vi "Heartbeat Reset.vi"(8 "error in":errorcluster, 10 "CANopen Message":refnum<class "CANopen Response Message.lvclass">, 11 "CANopen Master in":refnum<class "CANopen Master.lvclass">) -> (0 "error out":errorcluster, 3 "CANopen Master out":refnum<class "CANopen Master.lvclass">)   [LabVIEW 2024, in "CANopen Master.lvlib" / "CANopen Master.lvclass"]
uses:
  CANopen Master.lvclass
  CANopen Master.lvclass/CANopen Master.ctl
  Heartbeat/Heartbeat.lvclass
  Network Mangement/Network Mangement.lvclass
  CANopen Response/CANopen Response Message.lvclass
  D:/git/CANopen-XNET/CANopen Message/CANopen Message.lvclass
  D:/git/CANopen-XNET/CANopen Response/CANopen Response Message.lvclass
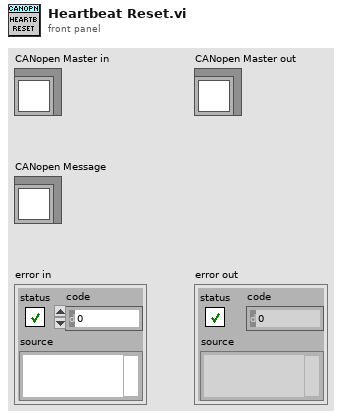
[diagram p1: front panel]
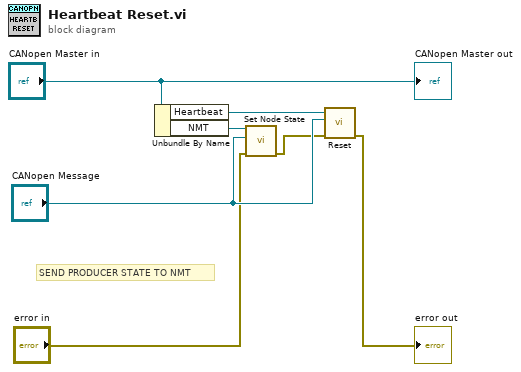
[diagram p0: block diagram]
diagram:
  # "SEND PRODUCER STATE TO NMT"
  n1 = Unbundle By Name("CANopen Master in") -> ("Heartbeat"=w6:refnum<class "Heartbeat.lvclass">, "NMT"=w4:refnum<class "Network Mangement.lvclass">)
  n2 = call "Set Node State.vi"("Error In"="error in", "CANopen Message"="CANopen Message", "reference in"=w4) -> ("Error Out"=w1:errorcluster)  [unwired: 7 in, 1 out]
  n3 = call "Reset.vi"("Error In"=w1, "CANopen Message"="CANopen Message", "reference in"=w6) -> ("Error Out"=→"error out":errorcluster)  [unwired: 7 in, 1 out]
  "CANopen Master out" <- "CANopen Master in"
